vi "TDMS.SetMetadata.vi"(8 "error in (no error)":errorcluster, 9 "DUTs":bool[](array[boolean])=[FALSE, FALSE, FALSE, FALSE, FALSE, FALSE, FALSE, FALSE, FALSE], 10 "LVTransitionParameters":T2={"ODH"={"Level"=1.0, "Band (+-)"=0.5, "TimeTolerance"=0.095}, "OPH_Duty"={"Level"=65.0, "Band (+-)"=10.0, "TimeTolerance"=0.095}, "OPH_Freq"={"Level"=100.0, "Band (+-)"=10.0, "TimeTolerance"=0.095}}, 11 "TestMetaData":T1) -> (0 "error out":errorcluster)   [LabVIEW 2014, in "NIAnalysis.lvlib"]
uses:
  NIAnalysis.lvlib
  Types/Public.LVAnalysis.ctl
  Types/Public.ChLVAnalysis.ctl
  Constants.vi
panel:
  in  "DUTs.SN":string[](array[string])
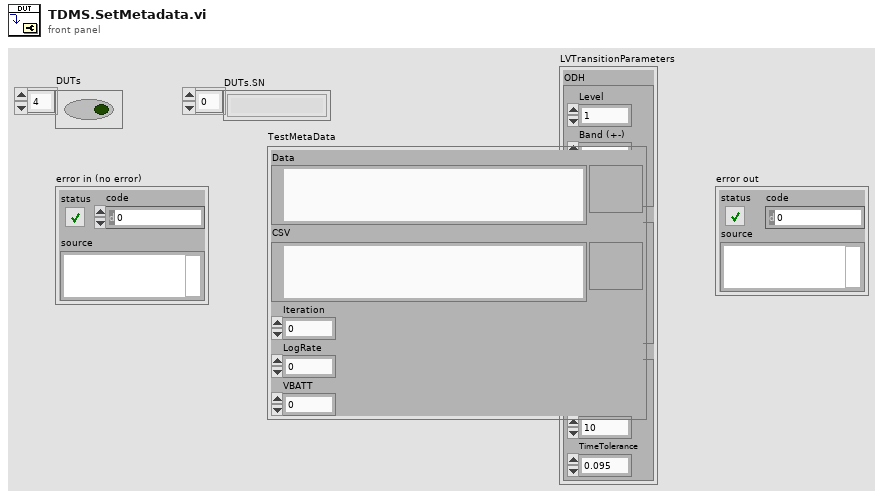
[diagram p1: front panel]
types:
  T1 = cluster{"Data":path, "CSV":path, "Iteration":i32, "LogRate":dbl, "VBATT":dbl}
  T2 = typedef "NIAnalysis.lvlib/Public.LVAnalysis.ctl" = cluster{"ODH":T3, "OPH_Duty":T3, "OPH_Freq":T3}
  T3 = typedef "NIAnalysis.lvlib/Public.ChLVAnalysis.ctl" = cluster{"Level":dbl, "Band (+-)":dbl, "TimeTolerance":dbl}
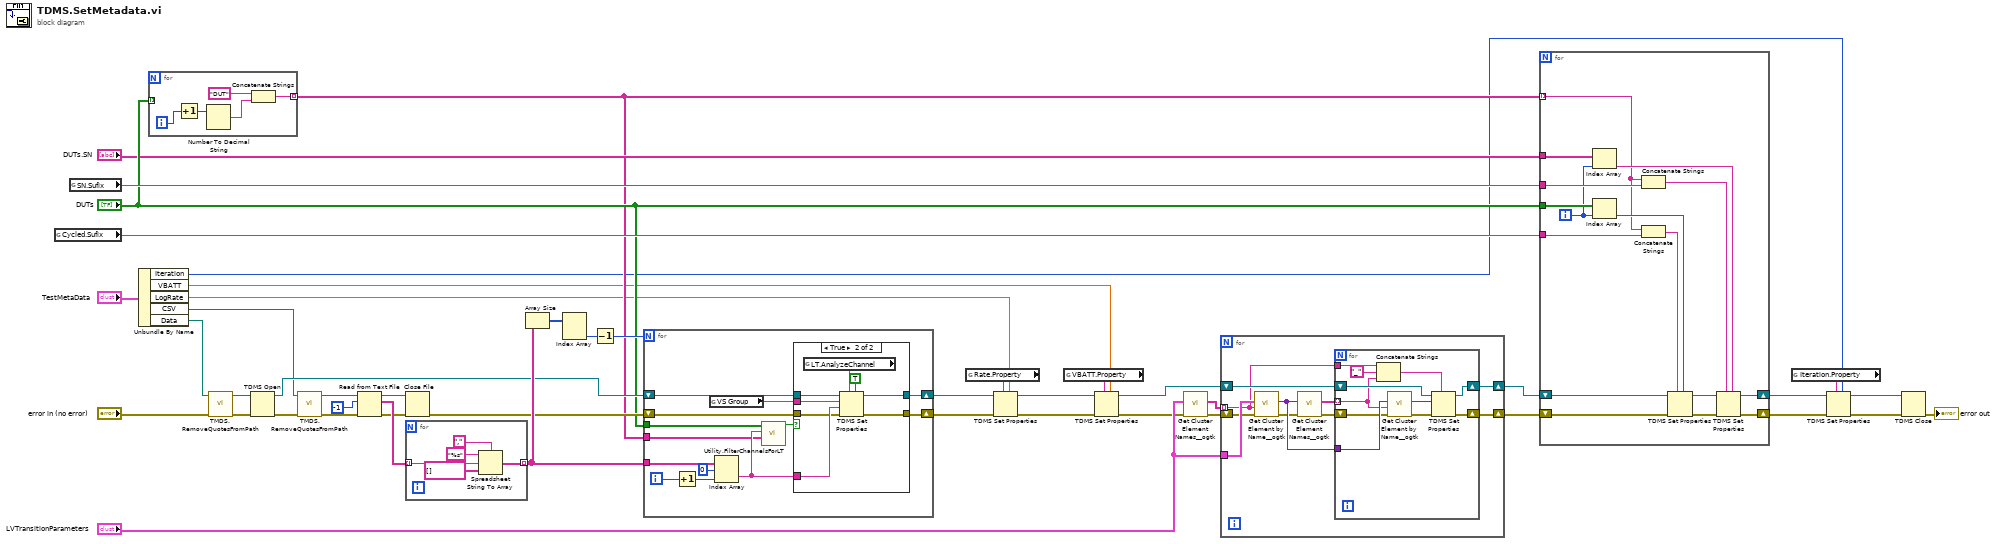
[diagram p0: block diagram]
diagram:
  n1 = global read "Constants.vi" "Cycled.Sufix"() -> (w45:string)
  n2 = global read "Constants.vi" "SN.Sufix"() -> (w44:string)
  n3 = Unbundle By Name("TestMetaData") -> ("Iteration"=w11:i32, "VBATT"=w10:dbl, "LogRate"=w9:dbl, "CSV"=w8:path, "Data"=w6:path)
  n4 = for {
    tunnel: "DUTs" -> [_] mode=indexing
    tunnel: [w47] -> w13 mode=indexing
    i -> [w48]
    n5 = Increment(x=w48) -> (x+1=w50:i32)
    n6 = Number To Decimal String(number=w50) -> (decimal integer string=w49:string)  [unwired: 1 in]
    n7 = Concatenate Strings("DUT", w49) -> (w47:string)
  }
  n8 = call "TMDS.RemoveQuotesFromPath.vi"("error in (no error)"="error in (no error)", "Data"=w6) -> ("error out"=w2:errorcluster, "Path"=w5:path)  [unwired: 8 in]
  n9 = TDMS Open(8:w2, 11:w5) -> (0:w4:errorcluster, 3:w25:refnum<k34>)  [unwired: 5 in]
  n10 = call "TMDS.RemoveQuotesFromPath.vi"("error in (no error)"=w4, "Data"=w8) -> ("error out"=w3:errorcluster, "Path"=w7:path)  [unwired: 8 in]
  n11 = Read from Text File(file (use dialog)=w7, count=-1, error in=w3) -> (refnum out=w31:refnum<file>, text=w32:string[], error out=w30:errorcluster)  [unwired: 1 in, 1 out]
  n12 = Close File(refnum=w31, error in=w30) -> (error out=w26:errorcluster)  [unwired: 1 out]
  n13 = for {
    tunnel: w32 -> [w56] mode=indexing
    tunnel: [w52] -> w27 mode=indexing
    n14 = Spreadsheet String To Array(delimiter (Tab)=",", format string="%s", spreadsheet string=w56, array type (2D Dbl)=string[] []) -> (array=w52:string[])
  }
  n15 = Array Size(array=w27) -> (size(s)=w34:i32[])
  n16 = Index Array(array=w34) -> (element #2=w33:i32)  [unwired: 2 in, 1 out]
  n17 = Decrement(x=w33) -> (x-1=w28:i32)
  n18 = for {
    N: w28 -> [_]
    tunnel: w27 -> [w67]
    tunnel: "DUTs" -> [w60]
    shift-right: [w65] -> w23
    shift-left: w25 -> [w64]
    shift-right: [w63] -> w24
    shift-left: w26 -> [w62]
    tunnel: w13 -> [w57]
    i -> [w68]
    n19 = Increment(x=w68) -> (x+1=w69:i32)
    n20 = global read "Constants.vi" "VS Group"() -> (w61:string)
    n21 = Index Array(array=w67, index (row)=0 ("disabled index (row)"), index (col)=w69) -> (element=w58:string)
    n22 = call "Utility.FilterChannelsForLT.vi"(9:"DUTs"=w57, "Channel"=w58, 11:"DUTs"=w60) -> ("Use?"=w59:bool)  [unwired: 7 in, 1 out]
    n23 = case shown="True" w59 {
      tunnel: w58 -> [_ w78]
      tunnel: [w71 w76] -> w65
      tunnel: w64 -> [w71 w75]
      tunnel: [w70 w74] -> w63
      tunnel: w62 -> [w70 w73]
      tunnel: w61 -> [_ w72]
      frame False {
      }
      frame True {
        n24 = global read "Constants.vi" "LT.AnalyzeChannel"() -> (w79:string)
        n25 = TDMS Set Properties(5:TRUE, 7:w79, 8:w73, 9:w78, 10:w72, 11:w75) -> (0:w74:errorcluster, 3:w76:refnum<k34>)  [unwired: 2 out]
      }
    }
  }
  n26 = global read "Constants.vi" "Rate.Property"() -> (w43:string)
  n27 = TDMS Set Properties(5:w9, 7:w43, 8:w24, 11:w23) -> (0:w22:errorcluster, 3:w21:refnum<k34>)  [unwired: 2 in, 2 out]
  n28 = global read "Constants.vi" "VBATT.Property"() -> (w35:string)
  n29 = TDMS Set Properties(5:w10, 7:w35, 8:w22, 11:w21) -> (0:w37:errorcluster, 3:w36:refnum<k34>)  [unwired: 2 in, 2 out]
  n30 = call <userlib>:"Get Cluster Element Names__ogtk.vi"("error in (no error)"=w37, "Cluster"="LVTransitionParameters") -> ("error out"=w38:errorcluster, "Element Names"=w40:string[])  [unwired: 8 in]
  n31 = for {
    shift-right: [w89] -> w42
    shift-left: w38 -> [w85]
    shift-right: [w87] -> w41
    shift-left: w36 -> [w88]
    tunnel: w40 -> [w80] mode=indexing
    tunnel: "LVTransitionParameters" -> [w86]
    n32 = call <userlib>:"Get Cluster Element by Name__ogtk.vi"("error in (no error)"=w85, "Element Name"=w80, "Cluster"=w86) -> ("error out"=w82:errorcluster, "VElement"=w84:variant)  [unwired: 6 in, 1 out]
    n33 = call <userlib>:"Get Cluster Element Names__ogtk.vi"("error in (no error)"=w82, "Cluster"=w84) -> ("error out"=w81:errorcluster, "Element Names"=w83:string[])  [unwired: 8 in]
    n34 = for {
      tunnel: w84 -> [w97]
      shift-right: [w98] -> w87
      shift-left: w88 -> [w99]
      shift-right: [w100] -> w89
      shift-left: w81 -> [w95]
      tunnel: w83 -> [w91] mode=indexing
      tunnel: w80 -> [w92]
      n35 = Concatenate Strings(w92, "_" ("string"), w91) -> (w90:string)
      n36 = call <userlib>:"Get Cluster Element by Name__ogtk.vi"("error in (no error)"=w95, "Element Name"=w91, "Cluster"=w97) -> ("error out"=w94:errorcluster, "VElement"=w96:variant)  [unwired: 6 in, 1 out]
      n37 = TDMS Set Properties(5:w96, 7:w90, 8:w94, 11:w99) -> (0:w100:errorcluster, 3:w98:refnum<k34>)  [unwired: 2 in, 2 out]
    }
  }
  n38 = for {
    tunnel: w45 -> [w116]
    shift-right: [w102] -> w18
    shift-left: w41 -> [w115]
    shift-right: [w103] -> w19
    shift-left: w42 -> [w114]
    tunnel: "DUTs" -> [w108]
    tunnel: w44 -> [w110]
    tunnel: "DUTs.SN" -> [w106]
    tunnel: w13 -> [w101] mode=indexing
    i -> [w104]
    n39 = Index Array(array=w106, index=w104) -> (element=w105:string)
    n40 = Index Array(array=w108, index=w104) -> (element=w107:bool)
    n41 = Concatenate Strings(w101, w110) -> (w109:string)
    n42 = Concatenate Strings(w101, w116) -> (w111:string)
    n43 = TDMS Set Properties(5:w107, 7:w111, 8:w114, 11:w115) -> (0:w113:errorcluster, 3:w112:refnum<k34>)  [unwired: 2 in, 2 out]
    n44 = TDMS Set Properties(5:w105, 7:w109, 8:w113, 11:w112) -> (0:w103:errorcluster, 3:w102:refnum<k34>)  [unwired: 2 in, 2 out]
  }
  n45 = global read "Constants.vi" "Iteration.Property"() -> (w20:string)
  n46 = TDMS Set Properties(5:w11, 7:w20, 8:w19, 11:w18) -> (0:w17:errorcluster, 3:w16:refnum<k34>)  [unwired: 2 in, 2 out]
  n47 = TDMS Close(8:w17, 11:w16) -> (0:→"error out":errorcluster)  [unwired: 1 out]
